vi "user input.vi"(8 "error in":errorcluster) -> (0 "error out":errorcluster, 3 "Inputs from system":T1)   [LabVIEW 2013, in "Custom Controller Module runtime.lvclass"]
uses:
  Custom Controller Module runtime.lvclass
  input user data.ctl
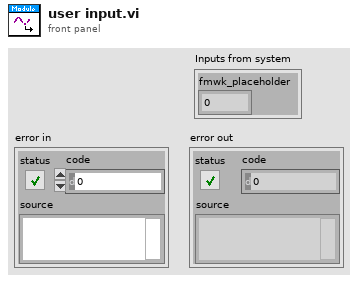
[diagram p1: front panel]
types:
  T1 = typedef "Custom Controller Module runtime.lvclass/input user data.ctl" = cluster{"fmwk_placeholder":i32}
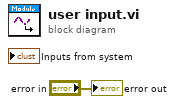
[diagram p0: block diagram]
diagram:
  "error out" <- "error in"
